vi "Generate Scan Coordinates.vi"(7 "Scan Pattern":T1(ring), 10 "Y Axis":T2, 11 "X Axis":T2) -> (1 "Array":cluster{"X":dbl, "Y":dbl}[](array[cluster]), 2 "Y Scale":dbl[](array[numeric]), 3 "X Scale":dbl[](array[numeric]))   [LabVIEW 2018]
uses:
  <vilib>/Analysis/1siggen.llb/Ramp Pattern by Samples.vi
  <vilib>/Analysis/NI_AALBase.lvlib
panel:
  out "XY Graph":cluster{"X":dbl, "Y":dbl}[](graph)
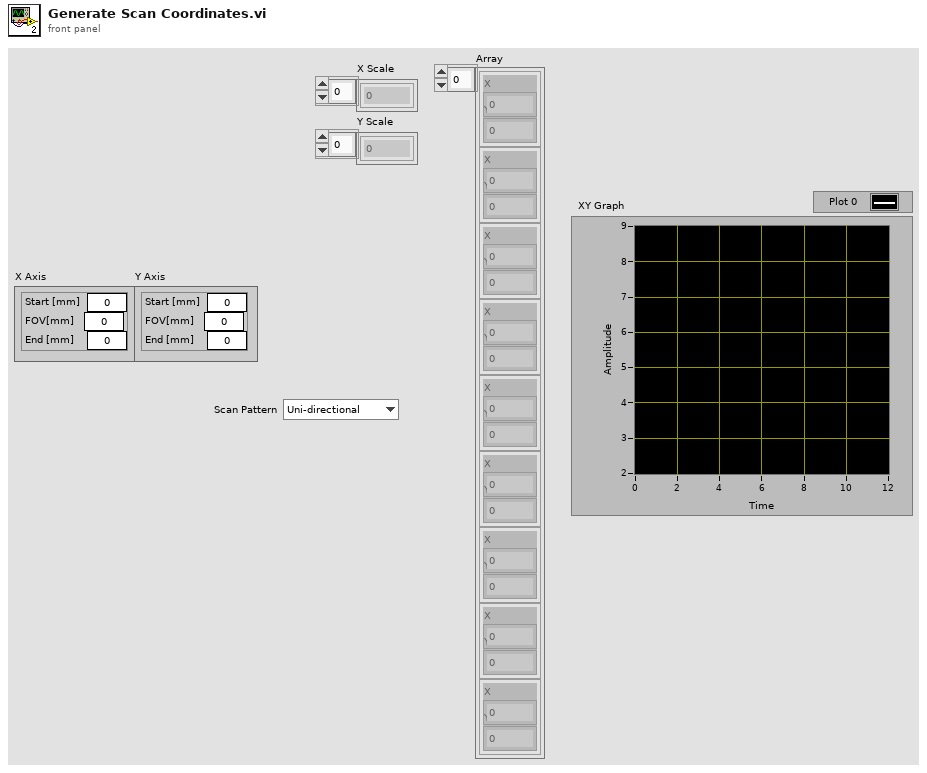
[diagram p1: front panel]
types:
  T1 = enum16{"Uni-directional", "Bi-Directional", "Spiral Out", "Spiral In"}
  T2 = cluster{"Start [mm]":dbl, "FOV[mm]":dbl, "End [mm]":dbl}
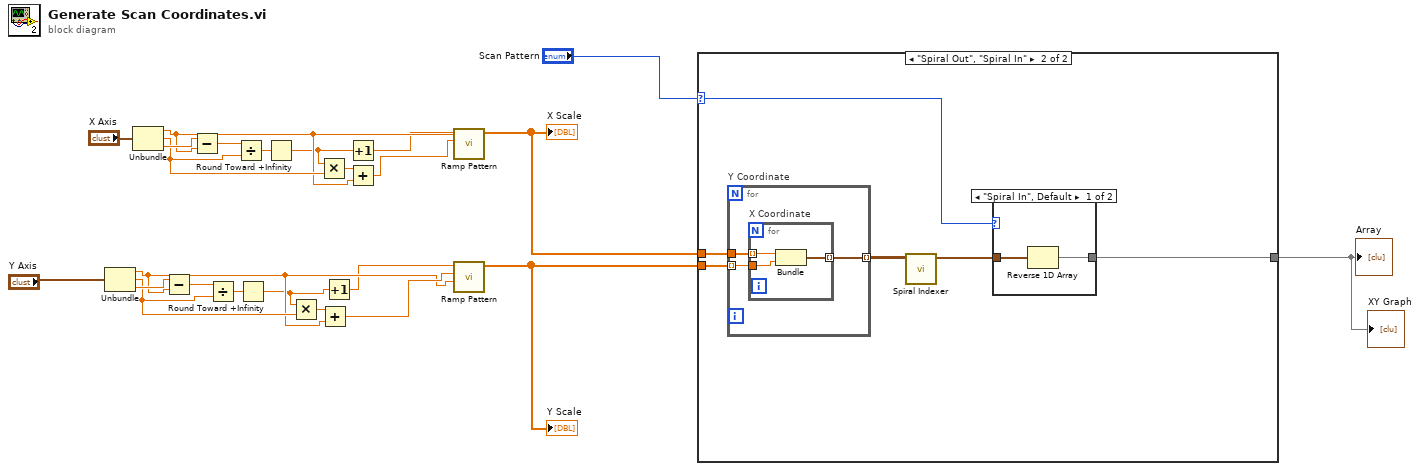
[diagram p0: block diagram]
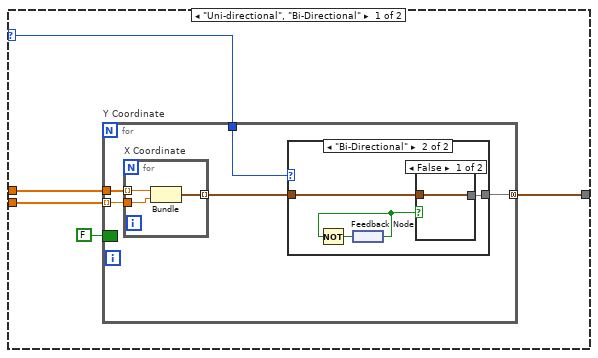
[diagram p2: hidden frame]
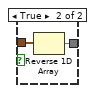
[diagram p4: hidden frame]
diagram:
  n1 = Unbundle("Y Axis") -> ("Start [mm]"=w5:dbl, "FOV[mm]"=w9:dbl, "End [mm]"=w12:dbl)
  n2 = Unbundle("X Axis") -> ("Start [mm]"=w14:dbl, "FOV[mm]"=w16:dbl, "End [mm]"=w19:dbl)
  n3 = Subtract(x=w12, y=w5) -> (x-y=w11:dbl)
  n4 = Subtract(x=w19, y=w14) -> (x-y=w18:dbl)
  n5 = Divide(x=w11, y=w9) -> (x/y=w10:dbl)
  n6 = Divide(x=w18, y=w16) -> (x/y=w17:dbl)
  n7 = Round Toward +Infinity(x=w10) -> (ceil(x): smallest int >= x=w2:dbl)
  n8 = Round Toward +Infinity(x=w17) -> (ceil(x): smallest int >= x=w4:dbl)
  n9 = Multiply(x=w2, y=w9) -> (x*y=w8:dbl)
  n10 = Multiply(x=w4, y=w16) -> (x*y=w15:dbl)
  n11 = Add(x=w8, y=w5) -> (x+y=w6:dbl)
  n12 = Increment(x=w2) -> (x+1=w1:dbl)
  n13 = Increment(x=w4) -> (x+1=w3:dbl)
  n14 = Add(x=w15, y=w14) -> (x+y=w13:dbl)
  n15 = call-poly <vilib>:"Ramp Pattern.vi"("start"=w14, "end"=w13, "samples"=w3) -> ("Ramp Pattern"=w23:dbl[])  [unwired: 7 in, 1 out]
  "X Scale" <- w23
  n16 = call-poly <vilib>:"Ramp Pattern.vi"("start"=w5, "end"=w6, "samples"=w1) -> ("Ramp Pattern"=w22:dbl[])  [unwired: 7 in, 1 out]
  "Y Scale" <- w22
  n17 = case shown="\"Spiral Out\", \"Spiral In\"" "Scan Pattern" {
    selector: "Scan Pattern" -> [w25 w48]
    tunnel: w23 -> [w29 w51]
    tunnel: w22 -> [w28 w50]
    tunnel: [w27 w47] -> w20
    frame "Uni-directional", "Bi-Directional" {
      n18 = for "Y Coordinate" {
        tunnel: w29 -> [w34]
        tunnel: w28 -> [w33] mode=indexing
        tunnel: [w30] -> w27 mode=concatenating
        tunnel: w25 -> [w32]
        border: FALSE -> [_]
        n19 = for "X Coordinate" {
          tunnel: w34 -> [w45] mode=indexing
          tunnel: w33 -> [w44]
          tunnel: [w43] -> w31 mode=indexing
          n20 = Bundle(w45, w44) -> (w43:cluster{dbl, dbl})  [unwired: 1 in]
        }
        n21 = case shown="\"Bi-Directional\"" w32 {
          tunnel: w31 -> [w35 w37]
          tunnel: [w35 w38] -> w30
          frame "Uni-directional", Default {
          }
          frame "Bi-Directional" {
            n22 = feedback #1() -> (w36:bool)
            n23 = Not(x=w36) -> (.not. x?=w39:bool)
            n24 = feedback-in #1(w39) -> ()
            n25 = case shown="False" w36 {
              tunnel: [w40 w42] -> w38
              tunnel: w37 -> [w40 w41]
              frame False {
              }
              frame True {
                n26 = Reverse 1D Array(array=w41) -> (reversed array=w42:cluster{dbl, dbl}[])
              }
            }
          }
        }
      }
    }
    frame "Spiral Out", "Spiral In" {
      n27 = for "Y Coordinate" {
        tunnel: w51 -> [w57]
        tunnel: w50 -> [w56] mode=indexing
        tunnel: [w55] -> w49 mode=indexing
        n28 = for "X Coordinate" {
          tunnel: w57 -> [w60] mode=indexing
          tunnel: w56 -> [w59]
          tunnel: [w58] -> w55 mode=indexing
          n29 = Bundle(w60, w59) -> (w58:cluster{dbl, dbl})  [unwired: 1 in]
        }
      }
      n30 = call "Spiral Indexer.vi"("Array 2"=w49) -> ("Array"=w46:cluster{dbl, dbl}[])  [unwired: 10 in]
      n31 = case shown="\"Spiral In\", Default" w48 {
        tunnel: [w52 w54] -> w47
        tunnel: w46 -> [w53 w54]
        frame "Spiral In", Default {
          n32 = Reverse 1D Array(array=w53) -> (reversed array=w52:cluster{dbl, dbl}[])
        }
        frame "Spiral Out" {
        }
      }
    }
  }
  "Array" <- w20
  "XY Graph" <- w20
